vi "delay.vi"(10 "Wait":dbl, 11 "In":bool) -> (3 "Out":bool)   [LabVIEW 2013]
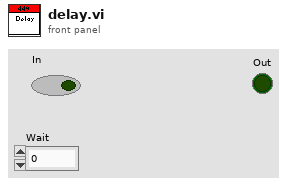
[diagram p1: front panel]
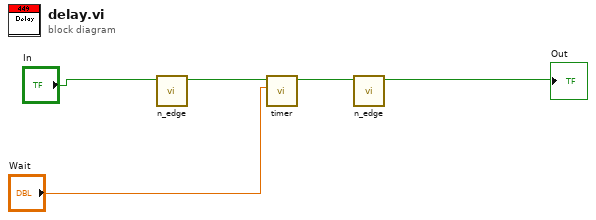
[diagram p0: block diagram]
diagram:
  n1 = call "n_edge.vi"("In"="In") -> ("Out"=w4:bool)  [unwired: 10 in]
  n2 = call "timer.vi"("Time"="Wait", "Set"=w4) -> ("Out"=w2:bool)  [unwired: 9 in]
  n3 = call "n_edge.vi"("In"=w2) -> ("Out"=→"Out":bool)  [unwired: 10 in]
